vi "Read_and_Write_Manipulator.vi"(5 "additional waiting time (0)":u32, 6 "Print?":bool, 7 "Motor":u16(ring) items=["none", "1", "2", "3", "4", "all"], 8 "error in (no error)":errorcluster, 9 "Value":string, 10 "Command":T1, 11 "VISA resource name":refnum<visa-resource-name>) -> (0 "error out":errorcluster={"status"=FALSE, "code"=1073676294, "source"="VISA Read in write_read.vi"}, 1 "Transmitted String":string, 2 "Answer":string, 3 "VISA ressource out":refnum<visa-resource-name>, 4 "Command accepted":bool)   [LabVIEW 2018]
uses:
  MCode_LV_86/Set Parameter.ctl
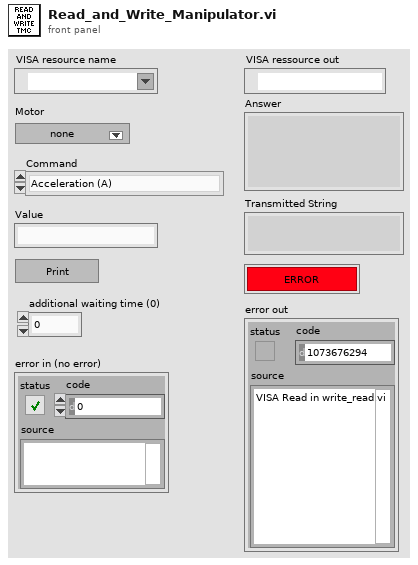
[diagram p1: front panel]
types:
  T1 = typedef "Set Parameter.ctl" = enum16{"Acceleration (A)", "Baud Rate (BD)", "Counter 1 (C1)", "Counter 2 (C2)", "Control C Software Reset (CE)", "Check Sum Enable (CK)", "Clock Mode (CM)", "Clock Mode Ratio (CR)", "Clock Mode Out Step Width (CW)", "Deceleration (D)", "Digital Filtering, Input 1 (D1)", "Digital Filtering, Input 2 (D2)", "Digital Filtering, Input 3 (D3)", "Digital Filtering, Input 4 (D4)", "Digital Filtering, Input 5 (D5)", "Digital Filtering, Input 9 (D9)", "Digital Filtering, Input 10 (D10)", "Digital Filtering, Input 11 (D11)", "Digital Filtering, Input 12 (D12)", "Deadband (DB)", "Decrement Variable (DC)", "Enable/Disable Drive (DE)", "Device Name (DN)", "End Program Execution (E)", "Encoder Function Enable (EE)", "Error Flag (EF)", "Encoder Lines (EL)", "Echo Mode (EM)", "Error Value (ER)", "Escape (ES)", "Execute Program at Address (EX)", "Firmware Version (VR)", "Hold (H)", "Hold Current (HC)", "Hold Current Delay Time (HI)", "Home to Encoder Index (HM)", "Home to Home Switch (HT)", "Increment Variable (IC)", "Initialize Parameters to NVM (IP)", "Input into Variable (IV)", "Jog Enable (JE)", "Limit Stop Mode (LM)", "Move Absolute (MA)", "Move Relative (MR)", "MicroStepping Select (MS)", "Motor Settling Delay Time (MT)", "Moving [Flag] (MV)", "Output 1 (O1)", "Output 2 (O2)", "Output 3 (O3)", "Output 4 (O4)", "Output 9 (O9)", "Output 10 (O10)", "Output 11 (O11)", "Output 12 (O12)", "Output High Byte (9-12) (OH)", "Output Low Byte (1-4) (OL)", "Output Total (1-4 and 9-12) (OT)", "Position (P)", "Position Maintenance (PM)", "Party Mode (PY)", "Register 1 (R1)", "Register 2 (R2)", "Register 3 (R3)", "Register 4 (R4)", "Reset Error(\\03)", "Run Current (RC)", "Stall Factor (SF)", "Slew (SL)", "Stall Mode Set (SM)", "Upgrade Firmware (UG)", "Velocity Initial (VI)", "Velocity Maximum (VM)", "Current1 (I1)", "Current2 (I2)", "Current3 (I3)", "Current4 (I4)", "Current5 (I5)", "Current6 (I6)", "Save (S)"}
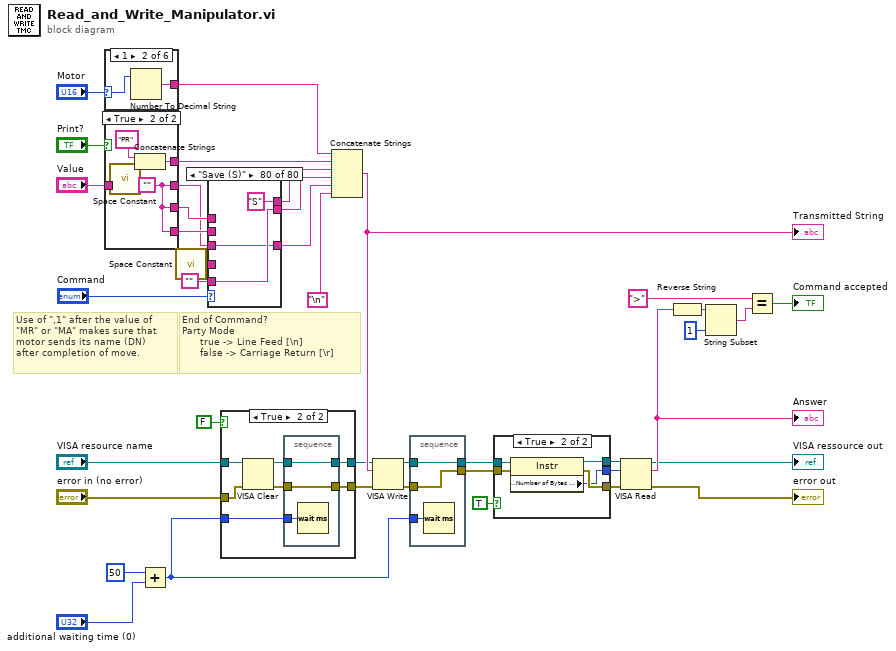
[diagram p0: block diagram]
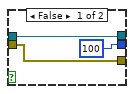
[diagram p3: hidden frame]
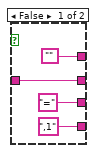
[diagram p4: hidden frame]
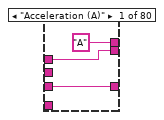
[diagram p5: hidden frame]
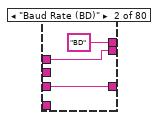
[diagram p6: hidden frame]
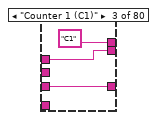
[diagram p7: hidden frame]
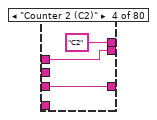
[diagram p8: hidden frame]
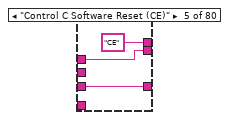
[diagram p9: hidden frame]
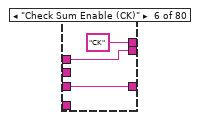
[diagram p10: hidden frame]
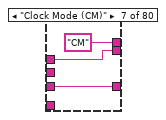
[diagram p11: hidden frame]
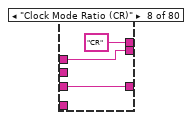
[diagram p12: hidden frame]
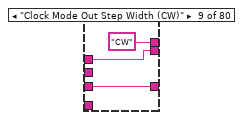
[diagram p13: hidden frame]
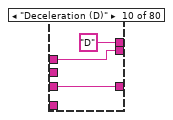
[diagram p14: hidden frame]
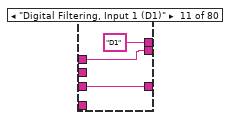
[diagram p15: hidden frame]
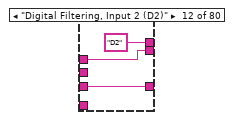
[diagram p16: hidden frame]
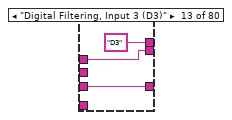
[diagram p17: hidden frame]
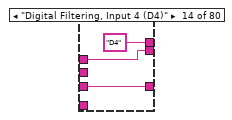
[diagram p18: hidden frame]
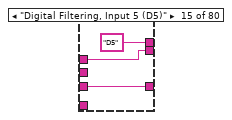
[diagram p19: hidden frame]
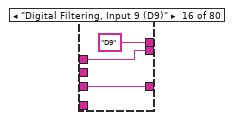
[diagram p20: hidden frame]
diagram:
  # "Use of \",1\" after the value of\n\"MR\" or \"MA\" makes sure that\nmotor sends its name (DN) \nafter completion of move."
  # "End of Command?\nParty Mode \n      true -> Line Feed [\\n]\n      false -> Carriage Return [\\r]"
  n1 = case shown="1" "Motor" {
    selector: "Motor" -> [_ w42 w44 w46 w48 _]
    tunnel: ["" w43 w45 w47 w49 "*"] -> w27
    frame 0, Default {
    }
    frame 1 {
      n2 = Number To Decimal String(number=w42) -> (decimal integer string=w43:string)  [unwired: 1 in]
    }
    frame 2 {
      n3 = Number To Decimal String(number=w44) -> (decimal integer string=w45:string)  [unwired: 1 in]
    }
    frame 3 {
      n4 = Number To Decimal String(number=w46) -> (decimal integer string=w47:string)  [unwired: 1 in]
    }
    frame 4 {
      n5 = Number To Decimal String(number=w48) -> (decimal integer string=w49:string)  [unwired: 1 in]
    }
    frame 5 {
    }
  }
  n6 = case shown="True" "Print?" {
    tunnel: ["" w57] -> w25
    tunnel: "Value" -> [w53 _]
    tunnel: [w53 w55] -> w10
    tunnel: ["=" w55] -> w12
    tunnel: [",1" w55] -> w11
    frame False {
    }
    frame True {
      w55 = ""
      n7 = call <vilib>:"Space Constant.vi"() -> ("String"=w58:string)
      n8 = Concatenate Strings("PR" ("string"), w58) -> (w57:string)
    }
  }
  n9 = Add(x=u32 50 ("milliseconds to wait"), y="additional waiting time (0)") -> (x+y=w4:u32)
  n10 = call <vilib>:"Space Constant.vi"() -> ("String"=w24:string)
  n11 = case shown="\"Save (S)\"" "Command" {
    tunnel: ["A" ("string") "BD" ("string") "C1" ("string") "C2" ("string") "CE" ("string") "CK" ("string") "CM" ("string") "CR" ("string") "CW" ("string") "D" ("string") "D1" ("string") "D2" ("string") "D3" ("string") "D4" ("string") "D5" ("string") "D9" ("string") "D10" ("string") "D11" ("string") "D12" ("string") "DB" ("string") "DC" ("string") "DE" ("string") "DN" ("string") "E" ("string") "EE" ("string") "EF" ("string") "EM" ("string") "ER" ("string") "ES" ("string") "EX" ("string") "VR" ("string") "H" ("string") "HC" ("string") "HI" ("string") "HM" ("string") "HT" ("string") "IC" ("string") "IP" ("string") "IV" ("string") "JE" ("string") "LM" ("string") "MA" ("string") "MR" ("string") "MS" ("string") "MT" ("string") "O1" ("string") "O2" ("string") "O3" ("string") "O4" ("string") "O9" ("string") "O10" ("string") "O11" ("string") "O12" ("string") "OH" ("string") "OL" ("string") "OT" ("string") "P" ("string") "PM" ("string") "PY" ("string") "R1" ("string") "R2" ("string") "R3" ("string") "R4" ("string") "RC" ("string") "SF" ("string") "SL" ("string") "SM" ("string") "UG" ("string") "VI" ("string") "VM" ("string") "EL" ("string") "\u0003" "MV" ("string") "I1" ("string") "I2" ("string") "I3" ("string") "I4" ("string") "I5" ("string") "I6" ("string") "S" ("string")] -> w28
    tunnel: w12 -> [w60 w63 w66 w69 w72 w75 w78 w81 w84 w87 w90 w93 w96 w99 w102 w105 w108 w111 w114 w117 w120 w123 w126 _ w132 w135 w138 w141 w144 w147 _ _ w156 w159 w162 w165 w168 w171 w174 w177 w180 _ _ w193 w196 w199 w202 w205 w208 w211 w214 w217 w220 w223 w226 w229 w233 w235 w238 w241 w244 w247 w250 w253 w256 w259 w262 w265 w268 w271 w274 _ _ w282 w286 w288 w292 w295 w298 _]
    tunnel: w24 -> [_ _ _ _ _ _ _ _ _ _ _ _ _ _ _ _ _ _ _ _ _ _ _ _ _ _ _ _ _ _ _ _ _ _ _ _ _ _ _ _ _ w186 w191 _ _ _ _ _ _ _ _ _ _ _ _ _ _ _ _ _ _ _ _ _ _ _ _ _ _ _ _ _ _ _ _ _ _ _ _ _]
    tunnel: [w60 w63 w66 w69 w72 w75 w78 w81 w84 w87 w90 w93 w96 w99 w102 w105 w108 w111 w114 w117 w120 w123 w126 w129 w132 w135 w138 w141 w144 w147 w151 w153 w156 w159 w162 w165 w168 w171 w174 w177 w180 w186 w191 w193 w196 w199 w202 w205 w208 w211 w214 w217 w220 w223 w226 w229 w233 w235 w238 w241 w244 w247 w250 w253 w256 w259 w262 w265 w268 w271 w274 w278 w280 w282 w286 w288 w292 w295 w298 w301] -> w22
    tunnel: "" -> [_ _ _ _ _ _ _ _ _ _ _ _ _ _ _ _ _ _ _ _ _ _ _ w129 _ _ _ _ _ _ w151 w153 _ _ _ _ _ _ _ _ _ _ _ _ _ _ _ _ _ _ _ _ _ _ _ _ _ _ _ _ _ _ _ _ _ _ _ _ _ _ _ w278 w280 _ _ _ _ _ _ w301]
    tunnel: w11 -> [_ _ _ _ _ _ _ _ _ _ _ _ _ _ _ _ _ _ _ _ _ _ _ _ _ _ _ _ _ _ _ _ _ _ _ _ _ _ _ _ _ w183 w187 _ _ _ _ _ _ _ _ _ _ _ _ _ _ _ _ _ _ _ _ _ _ _ _ _ _ _ _ _ _ _ _ _ _ _ _ _]
    tunnel: w10 -> [w59 w62 w65 w68 w71 w74 w77 w80 w83 w86 w89 w92 w95 w98 w101 w104 w107 w110 w113 w116 w119 w122 w125 w128 w131 w134 w137 w140 w143 w146 w149 w152 w155 w158 w161 w164 w167 w170 w173 w176 w179 w185 w188 w192 w195 w198 w201 w204 w207 w210 w213 w216 w219 w222 w225 w228 w231 w234 w237 w240 w243 w246 w249 w252 w255 w258 w261 w264 w267 w270 w273 w276 w281 w284 w285 w289 w291 w294 w297 w300]
    tunnel: [w59 w62 w65 w68 w71 w74 w77 w80 w83 w86 w89 w92 w95 w98 w101 w104 w107 w110 w113 w116 w119 w122 w125 w128 w131 w134 w137 w140 w143 w146 w149 w152 w155 w158 w161 w164 w167 w170 w173 w176 w179 w182 w189 w192 w195 w198 w201 w204 w207 w210 w213 w216 w219 w222 w225 w228 w231 w234 w237 w240 w243 w246 w249 w252 w255 w258 w261 w264 w267 w270 w273 w276 w281 w284 w285 w289 w291 w294 w297 w300] -> w9
    frame "Acceleration (A)" {
    }
    frame "Baud Rate (BD)" {
    }
    frame "Counter 1 (C1)" {
    }
    frame "Counter 2 (C2)" {
    }
    frame "Control C Software Reset (CE)" {
    }
    frame "Check Sum Enable (CK)" {
    }
    frame "Clock Mode (CM)" {
    }
    frame "Clock Mode Ratio (CR)" {
    }
    frame "Clock Mode Out Step Width (CW)" {
    }
    frame "Deceleration (D)" {
    }
    frame "Digital Filtering, Input 1 (D1)" {
    }
    frame "Digital Filtering, Input 2 (D2)" {
    }
    frame "Digital Filtering, Input 3 (D3)" {
    }
    frame "Digital Filtering, Input 4 (D4)" {
    }
    frame "Digital Filtering, Input 5 (D5)" {
    }
    frame "Digital Filtering, Input 9 (D9)" {
    }
    frame "Digital Filtering, Input 10 (D10)" {
    }
    frame "Digital Filtering, Input 11 (D11)" {
    }
    frame "Digital Filtering, Input 12 (D12)" {
    }
    frame "Deadband (DB)" {
    }
    frame "Decrement Variable (DC)" {
    }
    frame "Enable/Disable Drive (DE)" {
    }
    frame "Device Name (DN)" {
    }
    frame "End Program Execution (E)" {
    }
    frame "Encoder Function Enable (EE)" {
    }
    frame "Error Flag (EF)" {
    }
    frame "Echo Mode (EM)" {
    }
    frame "Error Value (ER)" {
    }
    frame "Escape (ES)" {
    }
    frame "Execute Program at Address (EX)" {
    }
    frame "Firmware Version (VR)" {
    }
    frame "Hold (H)" {
    }
    frame "Hold Current (HC)" {
    }
    frame "Hold Current Delay Time (HI)" {
    }
    frame "Home to Encoder Index (HM)" {
    }
    frame "Home to Home Switch (HT)" {
    }
    frame "Increment Variable (IC)" {
    }
    frame "Initialize Parameters to NVM (IP)" {
    }
    frame "Input into Variable (IV)" {
    }
    frame "Jog Enable (JE)" {
    }
    frame "Limit Stop Mode (LM)" {
    }
    frame "Move Absolute (MA)" {
      n12 = Concatenate Strings(w185, w183) -> (w182:string)
    }
    frame "Move Relative (MR)" {
      n13 = Concatenate Strings(w188, w187) -> (w189:string)
    }
    frame "MicroStepping Select (MS)" {
    }
    frame "Motor Settling Delay Time (MT)" {
    }
    frame "Output 1 (O1)" {
    }
    frame "Output 2 (O2)" {
    }
    frame "Output 3 (O3)" {
    }
    frame "Output 4 (O4)" {
    }
    frame "Output 9 (O9)" {
    }
    frame "Output 10 (O10)" {
    }
    frame "Output 11 (O11)" {
    }
    frame "Output 12 (O12)" {
    }
    frame "Output High Byte (9-12) (OH)" {
    }
    frame "Output Low Byte (1-4) (OL)" {
    }
    frame "Output Total (1-4 and 9-12) (OT)" {
    }
    frame "Position (P)" {
    }
    frame "Position Maintenance (PM)" {
    }
    frame "Party Mode (PY)" {
    }
    frame "Register 1 (R1)" {
    }
    frame "Register 2 (R2)" {
    }
    frame "Register 3 (R3)" {
    }
    frame "Register 4 (R4)" {
    }
    frame "Run Current (RC)" {
    }
    frame "Stall Factor (SF)" {
    }
    frame "Slew (SL)" {
    }
    frame "Stall Mode Set (SM)" {
    }
    frame "Upgrade Firmware (UG)" {
    }
    frame "Velocity Initial (VI)" {
    }
    frame "Velocity Maximum (VM)" {
    }
    frame "Encoder Lines (EL)" {
    }
    frame "Reset Error(\\03)" {
    }
    frame "Moving [Flag] (MV)" {
    }
    frame "Current1 (I1)" {
    }
    frame "Current2 (I2)" {
    }
    frame "Current3 (I3)" {
    }
    frame "Current4 (I4)" {
    }
    frame "Current5 (I5)" {
    }
    frame "Current6 (I6)" {
    }
    frame "Save (S)" {
    }
  }
  n14 = case shown="True" FALSE {
    tunnel: "VISA resource name" -> [w304 w306]
    tunnel: [w304 w310] -> w5
    tunnel: w4 -> [_ w311]
    tunnel: "error in (no error)" -> [w303 w308]
    tunnel: [w303 w309] -> w2
    frame False {
    }
    frame True {
      n15 = VISA Clear(VISA resource name=w306, error in (no error)=w308) -> (VISA resource name out=w305:refnum<visa-resource-name>, error out=w307:errorcluster)
      n16 = stacked-sequence {
        tunnel: w305 -> [w314]
        tunnel: [w314] -> w310
        tunnel: w307 -> [w313]
        tunnel: [w313] -> w309
        tunnel: w311 -> [w312]
        frame #0 {
          n17 = Wait (ms)(milliseconds to wait=w312) -> ()  [unwired: 1 out]
        }
      }
    }
  }
  n18 = Concatenate Strings(w27, w25, w28, w22, w9, "\n") -> (w19:string)
  "Transmitted String" <- w19
  n19 = VISA Write(VISA resource name=w5, write buffer=w19, error in (no error)=w2) -> (VISA resource name out=w37:refnum<visa-resource-name>, error out=w35:errorcluster)  [unwired: 1 out]
  n20 = stacked-sequence {
    tunnel: w37 -> [w317]
    tunnel: [w317] -> w36
    tunnel: w35 -> [w316]
    tunnel: [w316] -> w34
    tunnel: w4 -> [w315]
    frame #0 {
      n21 = Wait (ms)(milliseconds to wait=w315) -> ()  [unwired: 1 out]
    }
  }
  n22 = case shown="True" TRUE {
    tunnel: [w319 w325] -> w40
    tunnel: [w320 w324] -> w39
    tunnel: [u32 100 ("Bytes at Port") w323] -> w38
    tunnel: w36 -> [w320 w322]
    tunnel: w34 -> [w319 w321]
    frame False {
    }
    frame True {
      n23 = property class="Instr"(reference=w322, error in=w321) -> (reference out=w324:refnum<visa-resource-name>, error out=w325:errorcluster, "Serial Settings:Number of Bytes at Serial Port"=w323:u32)
    }
  }
  n24 = VISA Read(VISA resource name=w39, byte count=w38, error in (no error)=w40) -> (VISA resource name out=→"VISA ressource out":refnum<visa-resource-name>, read buffer=w8:string, error out=→"error out":errorcluster)  [unwired: 1 out]
  "Answer" <- w8
  n25 = Reverse String(1:w8) -> (0:w32:string)
  n26 = String Subset(string=w32, length (rest)=1 ("length (rest)")) -> (substring=w16:string)  [unwired: 1 in]
  n27 = Equal?(x=">", y=w16) -> (x = y?=→"Command accepted":bool)
